vi "Enable Debug Mode.vi"(8 "error in (no error)":errorcluster, 10 "Enable Debug":bool, 11 "Actor in":refnum<class "Main Controller Actor.lvclass">) -> (0 "error out":errorcluster, 3 "Actor out":refnum<class "Main Controller Actor.lvclass">)   [LabVIEW 2015, in "Main Controller Actor.lvclass"]
uses:
  Main Controller Actor.lvclass
  Main Controller Actor.lvclass/Main Controller Actor.ctl
  Re-use Libraries/Utility/Utility.lvlib
panel:
  out "View Button NAmes":string[](array[string])
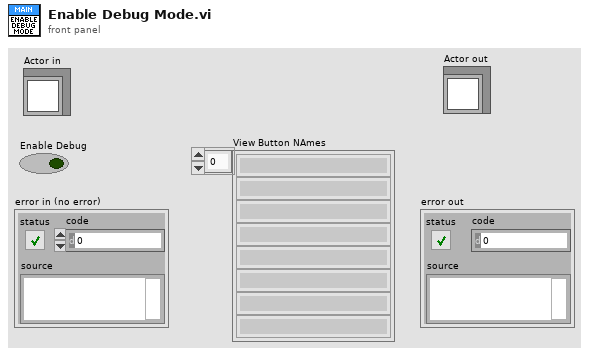
[diagram p1: front panel]
types:
  T1 = enum8{"Enabled", "Disabled", "Disabled and Grayed Out"}
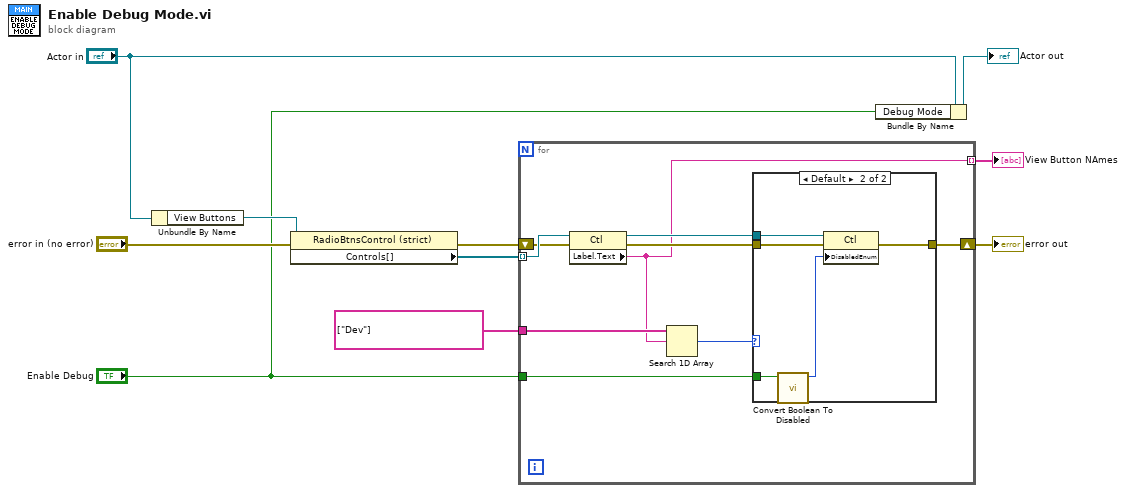
[diagram p0: block diagram]
diagram:
  n1 = Unbundle By Name("Actor in") -> ("View Buttons"=w10:refnum<vi>)
  n2 = property class="RadioBtnsControl (strict)"(reference=w10, error in="error in (no error)") -> (error out=w8:errorcluster, "Controls[]"=w9:refnum<vi>[])  [unwired: 1 out]
  n3 = for {
    tunnel: w9 -> [w19] mode=indexing
    shift-right: [w13] -> w5
    shift-left: w8 -> [w18]
    tunnel: string[] ["Dev"] -> [w17]
    tunnel: "Enable Debug" -> [w12]
    tunnel: [w11] -> w6 mode=indexing
    n4 = property class="Ctl"(reference=w19, error in=w18) -> (reference out=w14:refnum<vi>, error out=w15:errorcluster, "Label.Text"=w11:string)
    n5 = Search 1D Array(1D array=w17, element=w11) -> (index of element=w16:i32)  [unwired: 1 in]
    n6 = case shown="Default" w16 {
      tunnel: w15 -> [w20 w24]
      tunnel: w14 -> [_ w25]
      tunnel: [w20 w23] -> w13
      tunnel: w12 -> [_ w21]
      frame -1 {
      }
      frame Default {
        n7 = call "Convert Boolean To Disabled.vi"("Enabled"=w21) -> ("Disabled"=w22:T1)  [unwired: 10 in]
        n8 = property class="Ctl"(reference=w25, error in=w24, "DisabledEnum"=w22) -> (error out=w23:errorcluster)  [unwired: 1 out]
      }
    }
  }
  "error out" <- w5
  "View Button NAmes" <- w6
  n9 = Bundle By Name(cluster="Actor in", "Debug Mode"="Enable Debug") -> (→"Actor out":refnum<class "Main Controller Actor.lvclass">)
